vi "CheckArm.vi"() -> (2 "error out":errorcluster, 3 "read buffer":string)   [LabVIEW 2013]
panel:
  in  "rworks?":refnum<visa-resource-name>="GPIB0::20::INSTR"
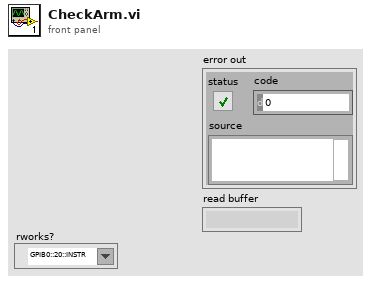
[diagram p1: front panel]
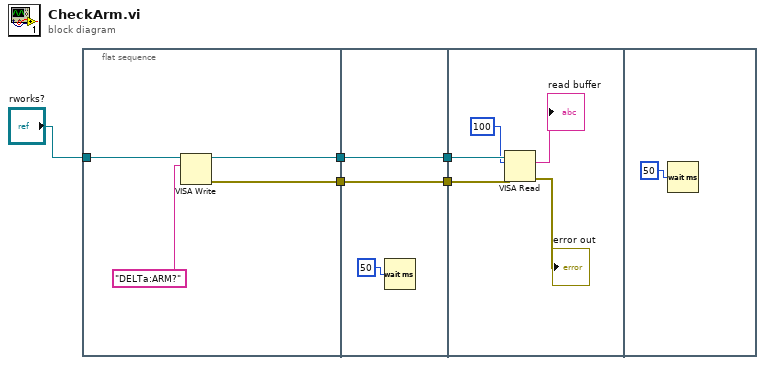
[diagram p0: block diagram]
diagram:
  n1 = flat-sequence {
    tunnel: [w9] -> w4
    tunnel: "rworks?" -> [w8]
    tunnel: [w7] -> w1
    tunnel: [w12] -> w5
    tunnel: w4 -> [w12]
    tunnel: [w11] -> w2
    tunnel: w1 -> [w11]
    tunnel: w5 -> [w17]
    tunnel: w2 -> [w15]
    frame #0 {
      n2 = VISA Write(VISA resource name=w8, write buffer="DELTa:ARM?") -> (VISA resource name out=w7:refnum<visa-resource-name>, error out=w9:errorcluster)  [unwired: 1 in, 1 out]
    }
    frame #1 {
      n3 = Wait (ms)(milliseconds to wait=50) -> ()  [unwired: 1 out]
    }
    frame #2 {
      n4 = VISA Read(VISA resource name=w15, byte count=100, error in (no error)=w17) -> (read buffer=→"read buffer":string, error out=→"error out":errorcluster)  [unwired: 2 out]
    }
    frame #3 {
      n5 = Wait (ms)(milliseconds to wait=50) -> ()  [unwired: 1 out]
    }
  }
